vi "AE75TX Set Curtailment.vi"(6 "Curtailment (%)":u16, 7 "Ramp Rate (kVA/s)":u16, 8 "error in":errorcluster, 10 "Modbus Configuration":T1, 11 "Modbus Master in":refnum<class "Modbus Master.lvclass">) -> (0 "error out":errorcluster, 3 "Modbus Master out":refnum<class "Modbus Master.lvclass">)   [LabVIEW 2018, in "AE75TX Actor.lvlib" / "AE75TX.lvclass"]
doc: "This VI handles setting curtailment and ramp rate for the AE75TX Inverter. <b>Ramp Rate</b> can be set between 1 and 50 kVA/s or 100 for maximum ramp rate. <b>Curtailment</b> can be set between 5 and 100 percent of total power rating."
uses:
  AE75TX.lvclass
  <vilib>/Modbus/master/Modbus Master.lvclass
  Controls/Modbus Configuration Cluster.ctl
  <vilib>/ORNL/CSEISMIC DDS/CSEISMIC DDS Base/Data Types/Controls/DeviceID.ctl
  <vilib>/ORNL/CSEISMIC DDS/CSEISMIC DDS Base/CSEISMIC DDS.lvclass
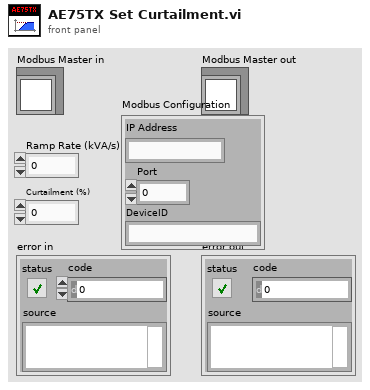
[diagram p1: front panel]
types:
  T1 = typedef "AE75TX Actor.lvlib/AE75TX.lvclass/Modbus Configuration Cluster.ctl" = cluster{"IP Address":string, "Port":u16, "DeviceID":T2}
  T2 = typedef "CSEISMIC DDS.lvlib/CSEISMIC DDS.lvclass/DeviceID.ctl" = string
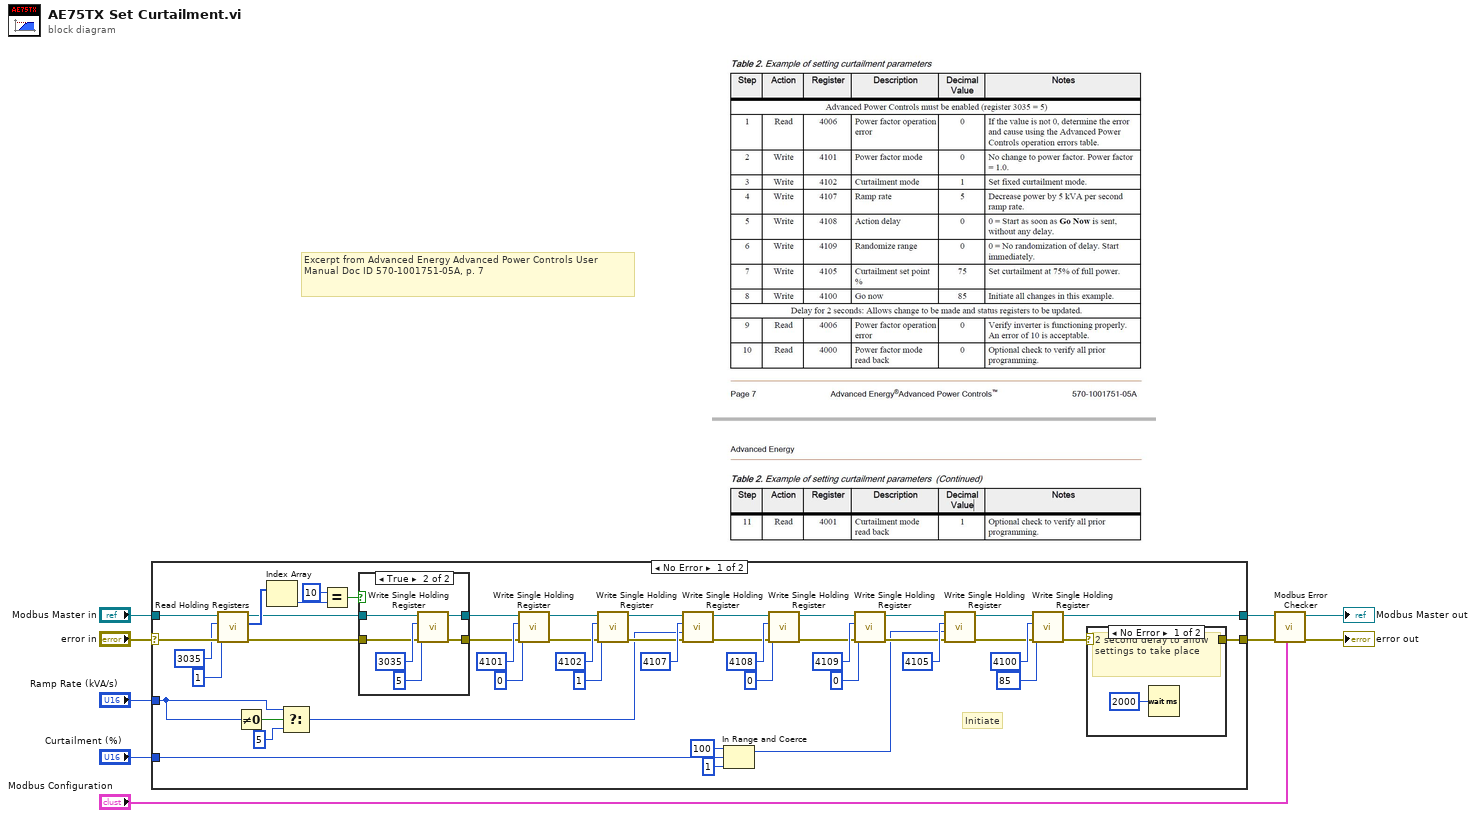
[diagram p0: block diagram]
diagram:
  # "Excerpt from Advanced Energy Advanced Power Controls User Manual Doc ID 570-1001751-05A, p. 7"
  n1 = case shown="No Error" "error in" {
    selector: "error in" -> [w27 w68]
    tunnel: "Modbus Master in" -> [w28 w69]
    tunnel: "Ramp Rate (kVA/s)" -> [w16 _]
    tunnel: "Curtailment (%)" -> [w13 _]
    tunnel: [w31 w69] -> w5
    tunnel: [w30 w68] -> w2
    frame No Error {
      # "Initiate"
      n2 = call-dynamic "Read Holding Registers.vi"("error in (no error)"=w27, "number of holding registers"=u16 1, "starting address"=u16 3035, "Modbus master in"=w28) -> ("error out"=w23:errorcluster, "register values"=w25:u16[], "Modbus master out"=w24:refnum<class "Modbus Master.lvclass">)  [unwired: 5 in]
      n3 = Not Equal To 0?(x=w16) -> (x != 0?=w15:bool)
      n4 = Index Array(array=w25) -> (element=w20:u16)  [unwired: 1 in]
      n5 = Select(t=w16, s=w15, f=u16 5) -> (s? t:f=w17:u16)
      n6 = Equal?(x=u16 10, y=w20) -> (x = y?=w18:bool)
      n7 = case shown="True" w18 {
        tunnel: w24 -> [w61 w65]
        tunnel: w23 -> [w60 w64]
        tunnel: [w60 w63] -> w22
        tunnel: [w61 w62] -> w21
        frame False {
        }
        frame True {
          n8 = call-dynamic "Write Single Holding Register.vi"("error in (no error)"=w64, "holding register value"=u16 5, "address"=u16 3035, "Modbus master in"=w65) -> ("error out"=w63:errorcluster, "Modbus master out"=w62:refnum<class "Modbus Master.lvclass">)  [unwired: 6 in]
        }
      }
      n9 = call-dynamic "Write Single Holding Register.vi"("error in (no error)"=w22, "holding register value"=u16 0, "address"=u16 4101, "Modbus master in"=w21) -> ("error out"=w52:errorcluster, "Modbus master out"=w51:refnum<class "Modbus Master.lvclass">)  [unwired: 6 in]
      n10 = call-dynamic "Write Single Holding Register.vi"("error in (no error)"=w52, "holding register value"=u16 1, "address"=u16 4102, "Modbus master in"=w51) -> ("error out"=w49:errorcluster, "Modbus master out"=w48:refnum<class "Modbus Master.lvclass">)  [unwired: 6 in]
      n11 = call-dynamic "Write Single Holding Register.vi"("error in (no error)"=w49, "holding register value"=w17, "address"=u16 4107, "Modbus master in"=w48) -> ("error out"=w43:errorcluster, "Modbus master out"=w42:refnum<class "Modbus Master.lvclass">)  [unwired: 6 in]
      n12 = In Range and Coerce(upper limit=u16 100, x=w13, lower limit=u16 1) -> (coerced(x)=w10:u16)  [unwired: 1 out]
      n13 = call-dynamic "Write Single Holding Register.vi"("error in (no error)"=w43, "holding register value"=u16 0, "address"=u16 4108, "Modbus master in"=w42) -> ("error out"=w40:errorcluster, "Modbus master out"=w41:refnum<class "Modbus Master.lvclass">)  [unwired: 6 in]
      n14 = call-dynamic "Write Single Holding Register.vi"("error in (no error)"=w40, "holding register value"=u16 0, "address"=u16 4109, "Modbus master in"=w41) -> ("error out"=w37:errorcluster, "Modbus master out"=w38:refnum<class "Modbus Master.lvclass">)  [unwired: 6 in]
      n15 = call-dynamic "Write Single Holding Register.vi"("error in (no error)"=w37, "holding register value"=w10, "address"=u16 4105, "Modbus master in"=w38) -> ("error out"=w33:errorcluster, "Modbus master out"=w34:refnum<class "Modbus Master.lvclass">)  [unwired: 6 in]
      n16 = call-dynamic "Write Single Holding Register.vi"("error in (no error)"=w33, "holding register value"=u16 85, "address"=u16 4100, "Modbus master in"=w34) -> ("error out"=w32:errorcluster, "Modbus master out"=w31:refnum<class "Modbus Master.lvclass">)  [unwired: 6 in]
      n17 = case shown="No Error" w32 {
        selector: w32 -> [w57 w59]
        tunnel: [w57 w59] -> w30
        frame No Error {
          # "2 second delay to allow settings to take place"
          n18 = Wait (ms)(milliseconds to wait=u32 2000) -> ()  [unwired: 1 out]
        }
        frame Error {
        }
      }
    }
    frame Error {
    }
  }
  n19 = call "Modbus Error Checker.vi"("Modbus Configuration"="Modbus Configuration", "error in"=w2, "Modbus Master in"=w5) -> ("error out"=→"error out":errorcluster, "Modbus Master out"=→"Modbus Master out":refnum<class "Modbus Master.lvclass">)  [unwired: 6 in, 1 out]
